vi "PV_Gnl_Counter.vi"(1 "Reset(F)":bool) -> (0 "Counter":u64)   [LabVIEW 2020]
doc: "Fonction :\n\nCette fonction renvoie son nombre d'exécution depuis sa première exécution ou depuis le dernier Reset."
panel:
  # "Input"
  # "Output"
  # "Local"
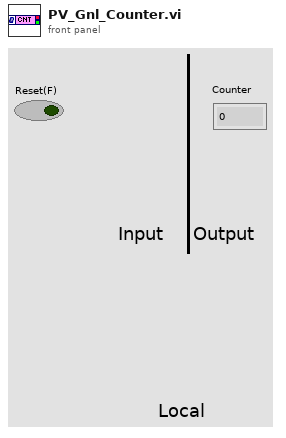
[diagram p1: front panel]
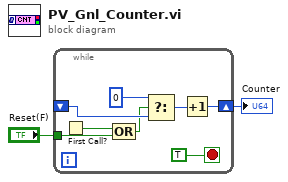
[diagram p0: block diagram]
diagram:
  n1 = while {
    shift-right: [w7] -> w2
    shift-left: _ -> [w6]
    tunnel: "Reset(F)" -> [w3]
    stop <- TRUE stop-if-true
    n2 = First Call?() -> (First Call?: T/F=w5:bool)
    n3 = Compound Arithmetic op=OR(w5, w3) -> (w4:bool)
    n4 = Select(t=u64 0, s=w4, f=w6) -> (s? t:f=w8:u64)
    n5 = Increment(x=w8) -> (x+1=w7:u64)
  }
  "Counter" <- w2
